vi "parseFA.vi"(8 "error in (no error)":errorcluster, 10 "ModbusBuffer in":refnum<class "ModbusBuffer.lvclass">, 11 "FAILC in":refnum<class "FAILC.lvclass">) -> (0 "error out":errorcluster, 1 "ParseSuccessful":bool, 2 "ModbusBuffer out":refnum<class "ModbusBuffer.lvclass">, 3 "FAILC out":refnum<class "FAILC.lvclass">)   [LabVIEW 2016, in "RTFAILC.lvlib" / "FAILC.lvclass"]
uses:
  FAILC.lvclass
  D:/Code/ts_M1M3Support/Common_RT_ILC/ILC/ILC.lvclass
  Common_RT_Modbus/ModbusBuffer/ModbusBuffer.lvclass
  Common_RT_Modbus/ModbusBuffer/ModbusBuffer.lvclass/ModbusBuffer.ctl
  Common_RT_ILC/ILC/ILC.lvclass/ILC.ctl
  FAILC.lvclass/FAILC.ctl
  Common_RT_ILC/ILC/parseReportServerIDFrame.vi
  Common_RT_ILC/ILC/parseReportServerIDError.vi
  Common_RT_ILC/ILC/parseReportServerStatusFrame.vi
  Common_RT_ILC/ILC/parseReportServerStatusError.vi
  Common_RT_ILC/ILC/parseModeFrame.vi
  Common_RT_ILC/ILC/parseModeError.vi
  Common_RT_ILC/ILC/parseTemporaryAddressFrame.vi
  Common_RT_ILC/ILC/parseTemporaryAddressError.vi
  Common_RT_ILC/ILC/parseADCScanRateFrame.vi
  Common_RT_ILC/ILC/parseADCScanRateError.vi
  Common_RT_ILC/ILC/parseADCOffsetSensitivityFrame.vi
  Common_RT_ILC/ILC/parseADCOffsetSensitivityError.vi
  Common_RT_ILC/ILC/parseResetFrame.vi
  Common_RT_ILC/ILC/parseResetError.vi
  Common_RT_ILC/ILC/parseReportCalibrationDataFrame.vi
  Common_RT_ILC/ILC/parseReportCalibrationDataError.vi
  Common_RT_Modbus/ModbusBuffer/calculateCRC.vi
  Common_RT_Modbus/ModbusBuffer/readCRC.vi
  Common_RT_Modbus/ModbusBuffer/readTimestamp.vi
  Common_RT_Modbus/ModbusBuffer/readEndOfFrame.vi
  Common_RT_Modbus/ModbusBuffer/readSGL.vi
  Common_RT_Modbus/ModbusBuffer/readInstructionByte.vi
  Common_RT_Modbus/ModbusBuffer/readU48.vi
  Common_RT_Modbus/ModbusBuffer/readString.vi
  Common_RT_Modbus/ModbusBuffer/readU16.vi
  Common_RT_Modbus/ModbusBuffer/readTimestampByte.vi
  Common_RT_ILC/ILC/ILC.lvclass
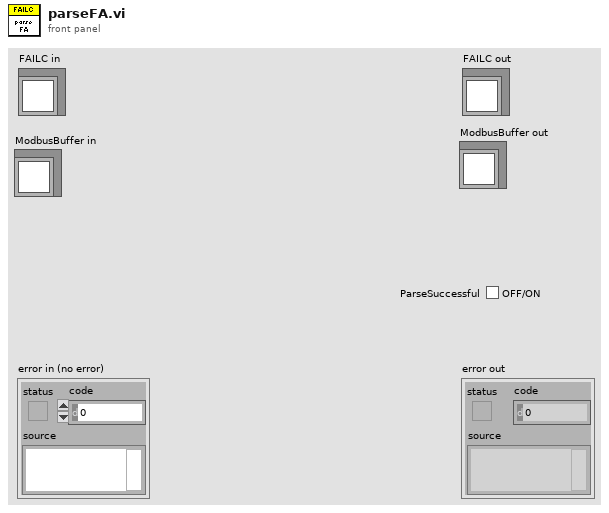
[diagram p1: front panel]
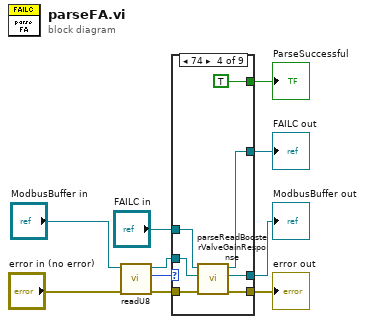
[diagram p0: block diagram]
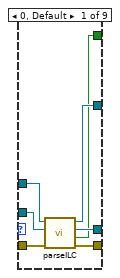
[diagram p2: hidden frame]
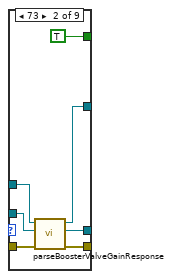
[diagram p3: hidden frame]
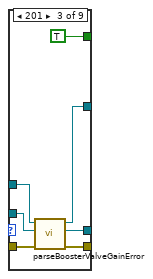
[diagram p4: hidden frame]
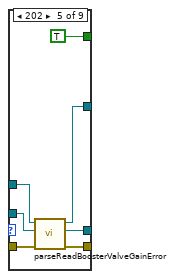
[diagram p5: hidden frame]
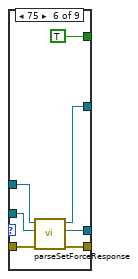
[diagram p6: hidden frame]
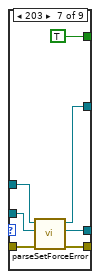
[diagram p7: hidden frame]
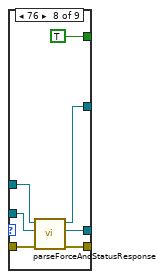
[diagram p8: hidden frame]
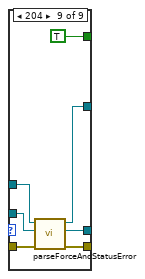
[diagram p9: hidden frame]
diagram:
  n1 = call "readU8.vi"("error in (no error)"="error in (no error)", "ModbusBuffer in"="ModbusBuffer in") -> ("error out"=w1:errorcluster, "Output"=w6:u8, "ModbusBuffer out"=w5:refnum<class "ModbusBuffer.lvclass">)  [unwired: 7 in]
  n2 = case shown="74" w6 {
    tunnel: "FAILC in" -> [w17 w24 w31 w38 w45 w52 w59 w66 w73]
    tunnel: w5 -> [w16 w23 w29 w35 w42 w51 w58 w65 w72]
    tunnel: [w14 w21 w30 w37 w44 w50 w57 w64 w71] -> w9
    tunnel: [w11 TRUE ("ParseSuccessful") TRUE ("ParseSuccessful") TRUE ("ParseSuccessful") TRUE ("ParseSuccessful") TRUE ("ParseSuccessful") TRUE ("ParseSuccessful") TRUE ("ParseSuccessful") TRUE ("ParseSuccessful")] -> w8
    tunnel: [w12 w22 w28 w36 w43 w49 w56 w63 w70] -> w3
    tunnel: [w13 w19 w25 w32 w40 w47 w54 w61 w68] -> w4
    tunnel: w1 -> [w15 w18 w26 w33 w39 w46 w53 w60 w67]
    frame 0, Default {
      n3 = call "parseILC.vi"("error in (no error)"=w15, "ModbusBuffer in"=w16, "ILC in"=w17) -> ("error out"=w12:errorcluster, "ParseSuccessful"=w11:bool, "ModbusBuffer out"=w13:refnum<class "ModbusBuffer.lvclass">, "ILC out"=w14:refnum<class "FAILC.lvclass">)  [unwired: 5 in]
    }
    frame 73 {
      n4 = call "parseBoosterValveGainResponse.vi"("error in (no error)"=w18, "ModbusBuffer in"=w23, "FAILC in"=w24) -> ("error out"=w22:errorcluster, "ModbusBuffer out"=w19:refnum<class "ModbusBuffer.lvclass">, "FAILC out"=w21:refnum<class "FAILC.lvclass">)  [unwired: 6 in]
    }
    frame 201 {
      n5 = call "parseBoosterValveGainError.vi"("error in (no error)"=w26, "ModbusBuffer in"=w29, "FAILC in"=w31) -> ("error out"=w28:errorcluster, "ModbusBuffer out"=w25:refnum<class "ModbusBuffer.lvclass">, "FAILC out"=w30:refnum<class "FAILC.lvclass">)  [unwired: 6 in]
    }
    frame 74 {
      n6 = call "parseReadBoosterValveGainResponse.vi"("error in (no error)"=w33, "ModbusBuffer in"=w35, "FAILC in"=w38) -> ("error out"=w36:errorcluster, "ModbusBuffer out"=w32:refnum<class "ModbusBuffer.lvclass">, "FAILC out"=w37:refnum<class "FAILC.lvclass">)  [unwired: 6 in]
    }
    frame 202 {
      n7 = call "parseReadBoosterValveGainError.vi"("error in (no error)"=w39, "ModbusBuffer in"=w42, "FAILC in"=w45) -> ("error out"=w43:errorcluster, "ModbusBuffer out"=w40:refnum<class "ModbusBuffer.lvclass">, "FAILC out"=w44:refnum<class "FAILC.lvclass">)  [unwired: 6 in]
    }
    frame 75 {
      n8 = call "parseSetForceResponse.vi"("error in (no error)"=w46, "ModbusBuffer in"=w51, "FAILC in"=w52) -> ("error out"=w49:errorcluster, "ModbusBuffer out"=w47:refnum<class "ModbusBuffer.lvclass">, "FAILC out"=w50:refnum<class "FAILC.lvclass">)  [unwired: 6 in]
    }
    frame 203 {
      n9 = call "parseSetForceError.vi"("error in (no error)"=w53, "ModbusBuffer in"=w58, "FAILC in"=w59) -> ("error out"=w56:errorcluster, "ModbusBuffer out"=w54:refnum<class "ModbusBuffer.lvclass">, "FAILC out"=w57:refnum<class "FAILC.lvclass">)  [unwired: 6 in]
    }
    frame 76 {
      n10 = call "parseForceAndStatusResponse.vi"("error in (no error)"=w60, "ModbusBuffer in"=w65, "FAILC in"=w66) -> ("error out"=w63:errorcluster, "ModbusBuffer out"=w61:refnum<class "ModbusBuffer.lvclass">, "FAILC out"=w64:refnum<class "FAILC.lvclass">)  [unwired: 6 in]
    }
    frame 204 {
      n11 = call "parseForceAndStatusError.vi"("error in (no error)"=w67, "ModbusBuffer in"=w72, "FAILC in"=w73) -> ("error out"=w70:errorcluster, "ModbusBuffer out"=w68:refnum<class "ModbusBuffer.lvclass">, "FAILC out"=w71:refnum<class "FAILC.lvclass">)  [unwired: 6 in]
    }
  }
  "error out" <- w3
  "FAILC out" <- w9
  "ParseSuccessful" <- w8
  "ModbusBuffer out" <- w4
